vi "Global Recipe.vi"() -> ()   [LabVIEW 2013]
panel:
  out "Recipe in Use":string[][](table)
  out "recipe name":string
  out "System Status :":u16(ring) items=["NOT READY", "E-STOPPED", "FAULTED", "PAUSING...", "PAUSED", "IDLE", "RUNNING", "UNCALIBRATED", "CALIBRATING...", "POWER OFF", "POWERING ON...", "MANUAL MODE", "CONNECTING..."]
  in  "Media Stop Button":bool
  in  "Pause Button":bool
  in  "Play Button":bool
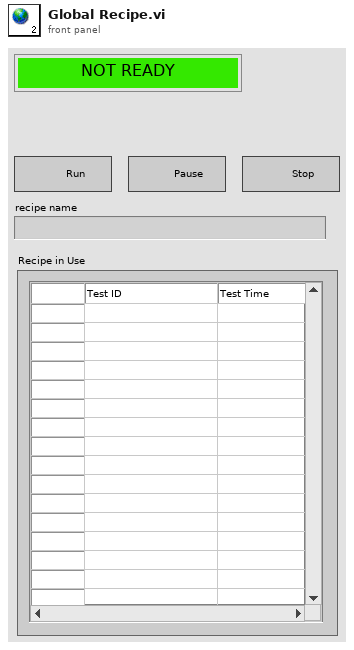
[diagram p1: front panel]
diagram:
